vi "caipirinha_subvi.vi"() -> (9 "sugar msg":string, 11 "sugar time":dbl, 13 "sugar qntity":dbl, 14 "rum quantity":dbl, 15 "rum time":dbl, 16 "rum msg":string, 17 "lime quantity":dbl, 18 "lime time":dbl, 19 "lime msg":string)   [LabVIEW 2019]
uses:
  <vilib>/Utility/file.llb/Read Delimited Spreadsheet (string).vi
panel:
  out "sugar":string
  out "lime":string
  out "rum":string
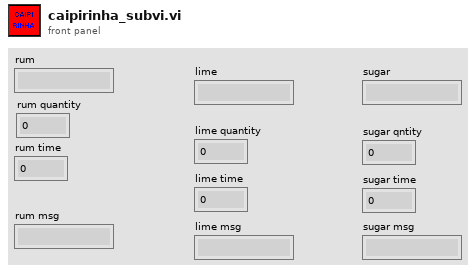
[diagram p1: front panel]
types:
  T1 = cluster{"first row[0]":string, "first row[1]":string, "first row[2]":string, "first row[3]":string, "first row[4]":string, "first row[5]":string, "first row[6]":string, "first row[7]":string, "first row[8]":string}
  T2 = cluster{"lime":string, "lime quantity":dbl, "lime time":dbl, "lime msg":string, "sugar":string, "sugar qntity":dbl, "sugar time":dbl, "sugar msg":string}
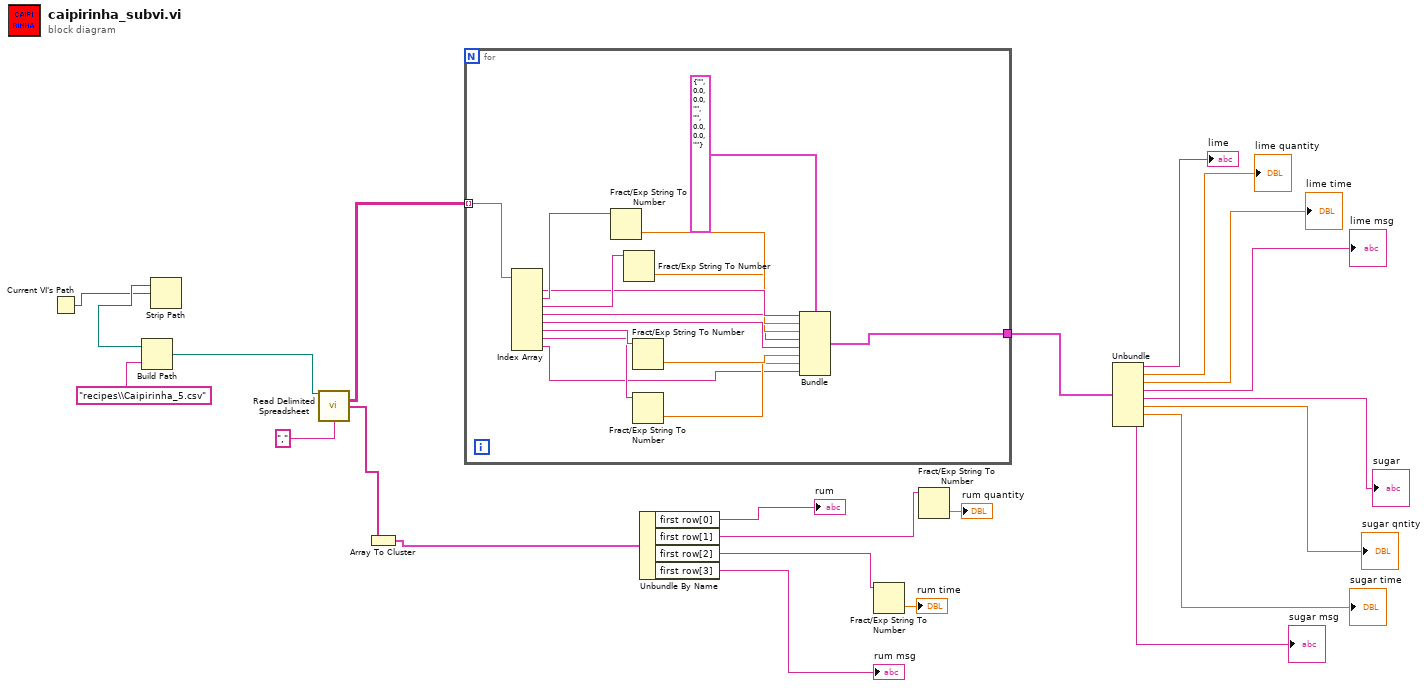
[diagram p0: block diagram]
diagram:
  n1 = Current VI's Path() -> (path=w2:path)
  n2 = Strip Path(path=w2) -> (stripped path=w4:path)  [unwired: 1 out]
  n3 = Build Path(base path=w4, name or relative path="recipes\\Caipirinha_5.csv") -> (appended path=w1:path)
  n4 = call-poly <vilib>:"Read Delimited Spreadsheet.vi"("file path (dialog if empty)"=w1, "delimiter (\\t)"="," ("delimiter (\\t)")) -> ("all rows"=w22:string[][], "first row"=w21:string[])  [unwired: 8 in, 4 out]
  n5 = Array To Cluster(array=w21) -> (cluster=w20:T1)
  n6 = for {
    tunnel: w22 -> [w38] mode=indexing
    tunnel: [w24] -> w13
    n7 = Index Array(array=w38) -> (element #1=w32:string, element #2=w37:string, element #3=w36:string, element #4=w29:string, element #5=w28:string, element #6=w35:string, element #7=w34:string, element #8=w25:string)  [unwired: 8 in]
    n8 = Fract/Exp String To Number(string=w37) -> (number=w31:dbl)  [unwired: 3 in, 1 out]
    n9 = Fract/Exp String To Number(string=w36) -> (number=w30:dbl)  [unwired: 3 in, 1 out]
    n10 = Fract/Exp String To Number(string=w35) -> (number=w27:dbl)  [unwired: 3 in, 1 out]
    n11 = Fract/Exp String To Number(string=w34) -> (number=w26:dbl)  [unwired: 3 in, 1 out]
    n12 = Bundle(cluster=T2 {"lime"="", "lime quantity"=0.0, "lime time"=0.0, "lime msg"="", "sugar"="", "sugar qntity"=0.0, "sugar time"=0.0, "sugar msg"=""} ("Cluster"), "lime"=w32, "lime quantity"=w31, "lime time"=w30, "lime msg"=w29, "sugar"=w28, "sugar qntity"=w27, "sugar time"=w26, "sugar msg"=w25) -> (w24:T2)
  }
  n13 = Unbundle By Name(w20) -> ("first row[0]"=→"rum":string, "first row[1]"=w19:string, "first row[2]"=w18:string, "first row[3]"=→"rum msg":string)
  n14 = Fract/Exp String To Number(string=w18) -> (number=→"rum time":dbl)  [unwired: 3 in, 1 out]
  n15 = Fract/Exp String To Number(string=w19) -> (number=→"rum quantity":dbl)  [unwired: 3 in, 1 out]
  n16 = Unbundle(w13) -> ("lime"=→"lime":string, "lime quantity"=→"lime quantity":dbl, "lime time"=→"lime time":dbl, "lime msg"=→"lime msg":string, "sugar"=→"sugar":string, "sugar qntity"=→"sugar qntity":dbl, "sugar time"=→"sugar time":dbl, "sugar msg"=→"sugar msg":string)
